vi "Measure.vi"(8 "error in (no error)":errorcluster, 11 "SMU in":refnum<class "NI SMU.lvclass">) -> (0 "error out":errorcluster, 2 "Data":variant, 3 "SMU out":refnum<class "NI SMU.lvclass">)   [LabVIEW 2020, in "NI SMU.lvlib" / "NI SMU.lvclass"]
uses:
  NI SMU.lvclass
  NI SMU.lvclass/NI SMU.ctl
  <instrlib>/niDCPower/nidcpower.llb/niDCPower Measurement Type.ctl
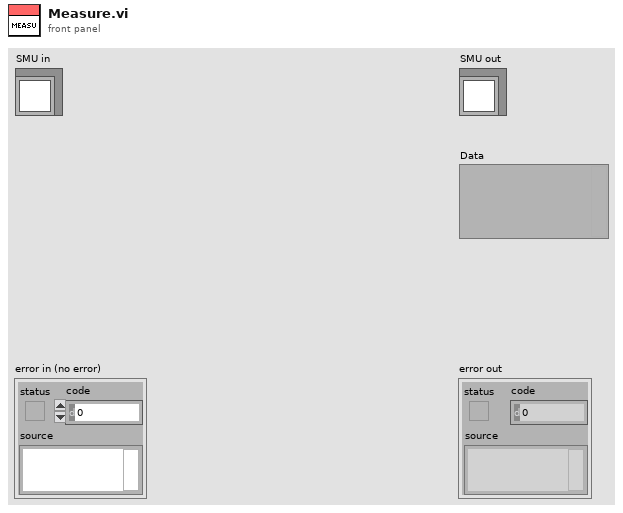
[diagram p1: front panel]
types:
  T1 = typedef "niDCPower Measurement Type.ctl" = i32
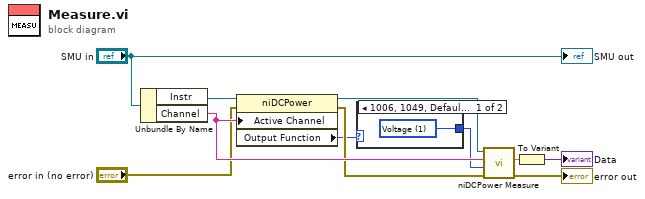
[diagram p0: block diagram]
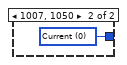
[diagram p2: hidden frame]
diagram:
  n1 = Unbundle By Name("SMU in") -> ("Instr"=w6:refnum<k15>, "Channel"=w7:string)
  n2 = property class="niDCPower"(reference=w6, error in="error in (no error)", "Active Channel"=w7) -> (reference out=w2:refnum<k15>, error out=w4:errorcluster, "Output Function"=w3:i32)
  n3 = case shown="1006, 1049, Default" w3 {
    tunnel: [w12 w13] -> w1
    frame 1006, 1049, Default {
      w12 = T1 1 items=["Current", "Voltage"] ("measurement type")
    }
    frame 1007, 1050 {
      w13 = T1 0 items=["Current", "Voltage"] ("measurement type")
    }
  }
  n4 = call <instrlib>:"niDCPower Measure.vi"("error in (no error)"=w4, "measurement type"=w1, "channel name"=w7, "instrument handle"=w2) -> ("error out"=→"error out":errorcluster, "measurement"=w9:dbl)  [unwired: 5 in, 1 out]
  n5 = To Variant(anything=w9) -> (Variant=→"Data":variant)
  "SMU out" <- "SMU in"
